vi "decode-33.vi"(0 "input string":string) -> (1 "数字 3":u32, 2 "x-y":u32, 3 "output data":i32, 4 "数字 2":u32)   [LabVIEW 2010]
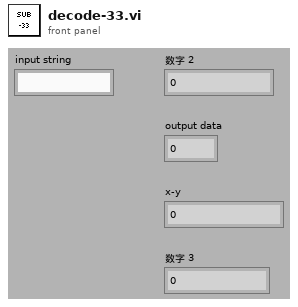
[diagram p1: front panel]
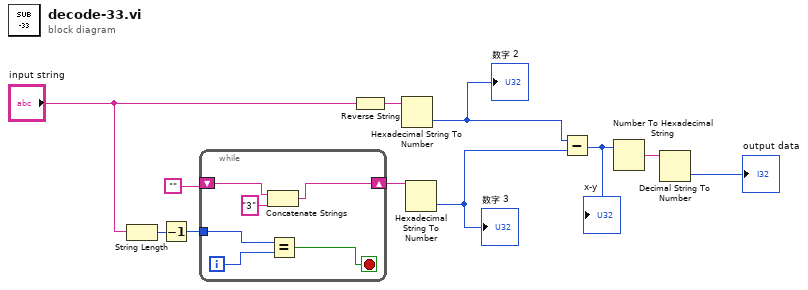
[diagram p0: block diagram]
diagram:
  n1 = String Length(string="input string") -> (length=w8:i32)
  n2 = Decrement(x=w8) -> (x-1=w10:i32)
  n3 = while {
    shift-right: [w16] -> w9
    shift-left: "" -> [w15]
    tunnel: w10 -> [w14]
    i -> [w13]
    stop <- w12 stop-if-true
    n4 = Concatenate Strings(w15, "3" ("字符串")) -> (w16:string)
    n5 = Equal?(x=w14, y=w13) -> (x = y?=w12:bool)
  }
  n6 = Reverse String(1:"input string") -> (0:w4:string)
  n7 = Hexadecimal String To Number(string=w4) -> (number=w1:u32)  [unwired: 2 in, 1 out]
  "数字 2" <- w1
  n8 = Hexadecimal String To Number(string=w9) -> (number=w2:u32)  [unwired: 2 in, 1 out]
  "数字 3" <- w2
  n9 = Subtract(x=w1, y=w2) -> (x-y=w3:u32)
  "x-y" <- w3
  n10 = Number To Hexadecimal String(2:w3) -> (0:w5:string)  [unwired: 1 in]
  n11 = Decimal String To Number(string=w5) -> (number=→"output data":i32)  [unwired: 2 in, 1 out]
